vi "Main Settings FG.vi"(6 "Action":enum8{"GET", "SET"}(ring), 8 "error in (no error)":errorcluster, 10 "Main Settings":T1={"RIO Device Address"="RIO0", "Local bitfile path"=path "", "RT bitfile path"=path "", "Number of injectors"=0}, 11 "Item Ref":T2 format="%.0x") -> (0 "error out":errorcluster, 2 "Main Settings out":T1, 3 "Item Ref out":T2=18446744073709551615 format="%.0x")   [LabVIEW 2019, in "Fuel Injector Analysis Addon Shared.lvlib"]
uses:
  Fuel Injector Analysis Addon Shared.lvlib
  <vilib>/NI VeriStand/Custom Device API/Custom Device Item Ref.ctl
  Types/Main Settings.ctl
  Constants.vi
  <vilib>/NI VeriStand/Custom Device API/Get Item Property (Path).vi
  <vilib>/NI VeriStand/Custom Device API/Get Item Property (String).vi
  <vilib>/NI VeriStand/Custom Device API/Get Item Property (U16).vi
  <vilib>/NI VeriStand/Custom Device API/Set Item Property (Path).vi
  <vilib>/NI VeriStand/Custom Device API/Set Item Property (String).vi
  <vilib>/NI VeriStand/Custom Device API/Set Item Property (U16).vi
  <vilib>/NI VeriStand/Custom Device API/Custom Device API.lvlib
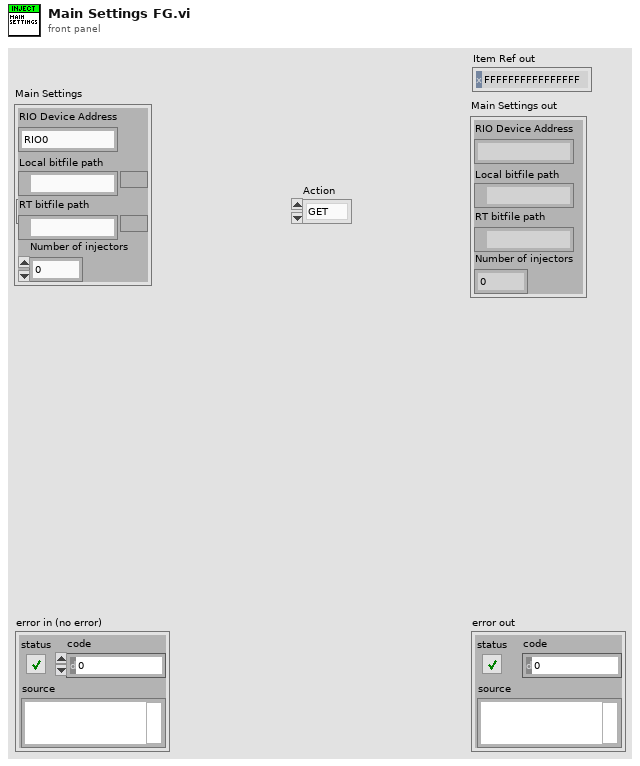
[diagram p1: front panel]
types:
  T1 = typedef "Fuel Injector Analysis Addon Shared.lvlib/Main Settings.ctl" = cluster{"RIO Device Address":string, "Local bitfile path":path, "RT bitfile path":path, "Number of injectors":u16}
  T2 = typedef "Custom Device API.lvlib/Custom Device Item Ref.ctl" = u64
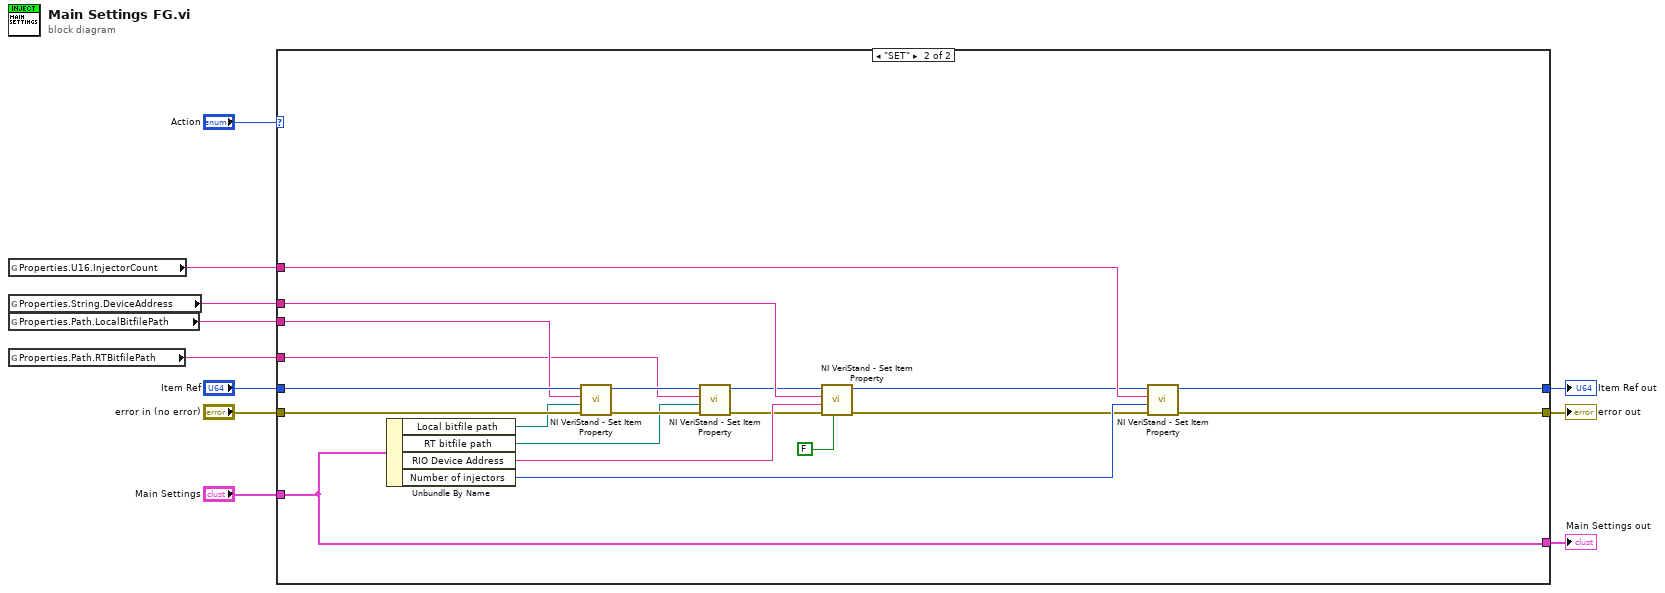
[diagram p0: block diagram]
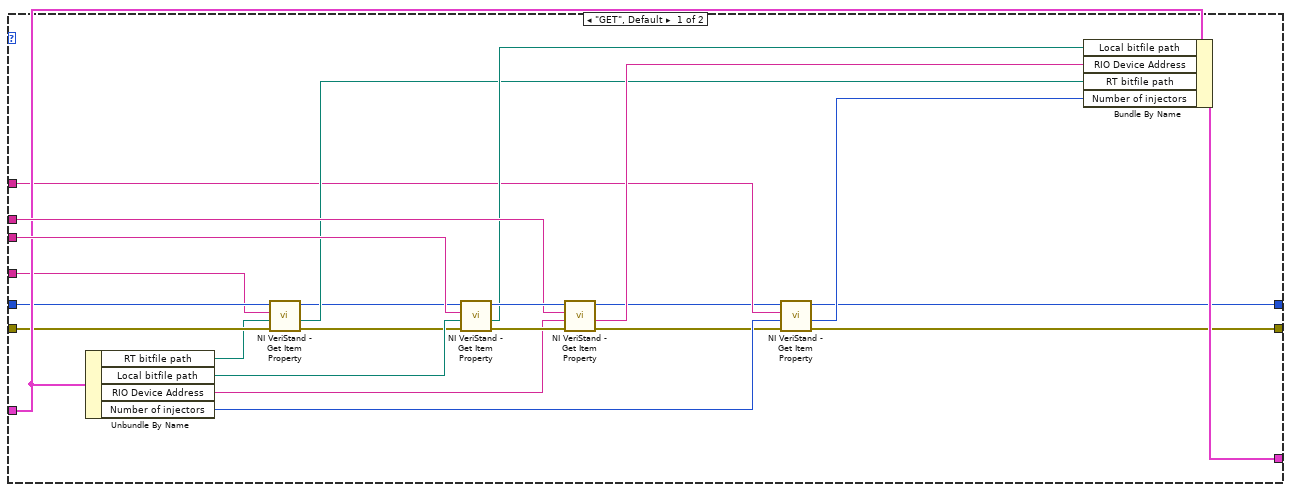
[diagram p2: hidden frame]
diagram:
  n1 = global read "Constants.vi" "Properties.U16.InjectorCount"() -> (w2:string)
  n2 = global read "Constants.vi" "Properties.String.DeviceAddress"() -> (w5:string)
  n3 = global read "Constants.vi" "Properties.Path.LocalBitfilePath"() -> (w4:string)
  n4 = global read "Constants.vi" "Properties.Path.RTBitfilePath"() -> (w3:string)
  n5 = case shown="\"SET\"" "Action" {
    tunnel: "error in (no error)" -> [w24 w55]
    tunnel: "Item Ref" -> [w25 w54]
    tunnel: "Main Settings" -> [w29 w52]
    tunnel: [w17 w39] -> w7
    tunnel: [w16 w38] -> w10
    tunnel: [w28 w52] -> w1
    tunnel: w4 -> [w35 w53]
    tunnel: w5 -> [w30 w49]
    tunnel: w3 -> [w23 w45]
    tunnel: w2 -> [w19 w41]
    frame "GET", Default {
      n6 = Unbundle By Name(w29) -> ("RT bitfile path"=w21:path, "Local bitfile path"=w32:path, "RIO Device Address"=w31:string, "Number of injectors"=w20:u16)
      n7 = call-poly <vilib>:"NI VeriStand - Get Item Property.vi"("error in (no error)"=w24, "Default Value"=w21, "Property Name"=w23, "Item Ref in"=w25) -> ("error out"=w15:errorcluster, "Value"=w22:path, "Item Ref out"=w14:T2)  [unwired: 4 in, 1 out]
      n8 = call-poly <vilib>:"NI VeriStand - Get Item Property.vi"("error in (no error)"=w15, "Default Value"=w32, "Property Name"=w35, "Item Ref in"=w14) -> ("error out"=w33:errorcluster, "Value"=w27:path, "Item Ref out"=w34:T2)  [unwired: 4 in, 1 out]
      n9 = call-poly <vilib>:"NI VeriStand - Get Item Property.vi"("error in (no error)"=w33, "Default Value"=w31, "Property Name"=w30, "Item Ref in"=w34) -> ("error out"=w13:errorcluster, "Value"=w26:string, "Item Ref out"=w12:T2)  [unwired: 4 in, 1 out]
      n10 = call-poly <vilib>:"NI VeriStand - Get Item Property.vi"("error in (no error)"=w13, "Default Value"=w20, "Property Name"=w19, "Item Ref in"=w12) -> ("error out"=w17:errorcluster, "Value"=w18:u16, "Item Ref out"=w16:T2)  [unwired: 4 in, 1 out]
      n11 = Bundle By Name(cluster=w29, "Local bitfile path"=w27, "RIO Device Address"=w26, "RT bitfile path"=w22, "Number of injectors"=w18) -> (w28:T1)
    }
    frame "SET" {
      n12 = Unbundle By Name(w52) -> ("Local bitfile path"=w46:path, "RT bitfile path"=w44:path, "RIO Device Address"=w50:string, "Number of injectors"=w40:u16)
      n13 = call-poly <vilib>:"NI VeriStand - Set Item Property.vi"("error in (no error)"=w55, "Value"=w46, "Property Name"=w53, "Item Ref in"=w54) -> ("error out"=w47:errorcluster, "Item Ref out"=w48:T2)  [unwired: 5 in, 1 out]
      n14 = call-poly <vilib>:"NI VeriStand - Set Item Property.vi"("error in (no error)"=w47, "Value"=w44, "Property Name"=w45, "Item Ref in"=w48) -> ("error out"=w43:errorcluster, "Item Ref out"=w42:T2)  [unwired: 5 in, 1 out]
      n15 = call-poly <vilib>:"NI VeriStand - Set Item Property.vi"("Binary String (T)"=FALSE, "error in (no error)"=w43, "Value"=w50, "Property Name"=w49, "Item Ref in"=w42) -> ("error out"=w37:errorcluster, "Item Ref out"=w36:T2)  [unwired: 4 in, 1 out]
      n16 = call-poly <vilib>:"NI VeriStand - Set Item Property.vi"("error in (no error)"=w37, "Value"=w40, "Property Name"=w41, "Item Ref in"=w36) -> ("error out"=w39:errorcluster, "Item Ref out"=w38:T2)  [unwired: 5 in, 1 out]
    }
  }
  "error out" <- w7
  "Item Ref out" <- w10
  "Main Settings out" <- w1
